vi "Voltage_to_unsigned_16bit_3.vi"(11 "Voltage_in":dbl) -> ()   [LabVIEW 2016]
panel:
  out "unsigned 8bit integer":u8
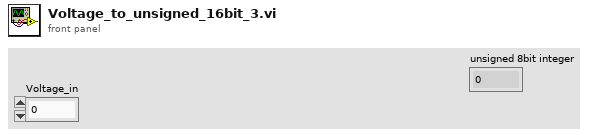
[diagram p1: front panel]
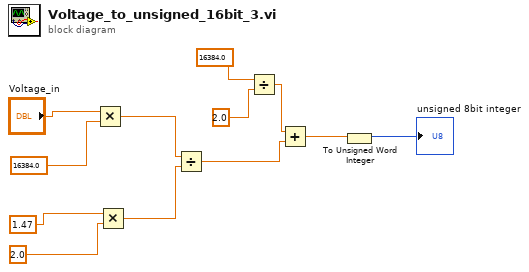
[diagram p0: block diagram]
diagram:
  n1 = Multiply(x="Voltage_in", y=16384.0) -> (x*y=w8:dbl)
  n2 = Multiply(x=1.47, y=2.0) -> (x*y=w7:dbl)
  n3 = Divide(x=w8, y=w7) -> (x/y=w3:dbl)
  n4 = Divide(x=16384.0, y=2.0) -> (x/y=w4:dbl)
  n5 = Add(x=w4, y=w3) -> (x+y=w1:dbl)
  n6 = To Unsigned Word Integer(number=w1) -> (unsigned 16bit integer=→"unsigned 8bit integer":u16)
